vi "测试参数读取.vi"(4 "error in (no error)":errorcluster caption="错误输入（无错误）", 6 "Container State":T5 caption="容器状态", 7 "Display State In":T1={"功能选择"=enum."扫描", "扫描参数"={"+ V"=1.0, "+ Δ V"=0.01, "+ limit I"=0.01, "- V"=1.0, "- Δ V"=0.01, "- limit I"=0.01, "NPLC"=1.0, "模型"=FALSE}, "保持时间"={"V"=0.1, "limit I"=0.01, "T"=10000.0, "ΔT"=1.0, "NPLC"=1.0}, "脉冲1"={"t0"=timestamp(0 s since 1904-01-01), "dt"=1.0, "Y"=[]}, "脉冲2"={"t0"=timestamp(0 s since 1904-01-01), "dt"=1.0, "Y"=[]}, "高速脉冲1"={"t0"=timestamp(0 s since 1904-01-01), "dt"=1.0, "Y"=[]}, "高速脉冲2"={"t0"=timestamp(0 s since 1904-01-01), "dt"=1.0, "Y"=[]}, "任意波形"={"t0"=timestamp(0 s since 1904-01-01), "dt"=1.0, "Y"=[]}} caption="显示状态输入" {"保持时间"."ΔT" min=0.5 max=100.0 step=0.1 format="%#_6ps"; "保持时间"."T" min=10.0 max=4294000.0 step=1.0 format="%#_6ps"; "保持时间"."NPLC" min=1.0 max=20.0 step=1.0; "保持时间"."limit I" min=1e-08 max=3.0 format="%#_6pA"; "保持时间"."V" min=-40.0 max=40.0 format="%#_6pV"; "扫描参数"."NPLC" min=0.001 max=25.0 step=0.001; "扫描参数"."- Δ V" min=5e-05 max=1.0 step=5e-05 format="%#_6pV"; "扫描参数"."+ Δ V" min=5e-05 max=1.0 step=5e-05 format="%#_6pV"; "扫描参数"."- V" min=-40.0 max=40.0 format="%#_6pV"; "扫描参数"."- limit I" min=1e-08 max=3.0 format="%#_6pA"; "扫描参数"."+ limit I" min=1e-08 max=3.0 format="%#_6pA"; "扫描参数"."+ V" min=-40.0 max=40.0 format="%#_6pV"}) -> (0 "error out":errorcluster caption="错误输出", 2 "Value":variant caption="值", 3 "Display State Out":T1={"功能选择"=enum."扫描", "扫描参数"={"+ V"=1.0, "+ Δ V"=0.01, "+ limit I"=0.01, "- V"=1.0, "- Δ V"=0.01, "- limit I"=0.01, "NPLC"=1.0, "模型"=FALSE}, "保持时间"={"V"=0.1, "limit I"=0.01, "T"=10000.0, "ΔT"=1.0, "NPLC"=1.0}, "脉冲1"={"t0"=timestamp(0 s since 1904-01-01), "dt"=1.0, "Y"=[]}, "脉冲2"={"t0"=timestamp(0 s since 1904-01-01), "dt"=1.0, "Y"=[]}, "高速脉冲1"={"t0"=timestamp(0 s since 1904-01-01), "dt"=1.0, "Y"=[]}, "高速脉冲2"={"t0"=timestamp(0 s since 1904-01-01), "dt"=1.0, "Y"=[]}, "任意波形"={"t0"=timestamp(0 s since 1904-01-01), "dt"=1.0, "Y"=[]}} caption="显示状态输出" {"保持时间"."ΔT" min=0.5 max=100.0 step=0.1 format="%#_6ps"; "保持时间"."T" min=10.0 max=4294000.0 step=1.0 format="%#_6ps"; "保持时间"."NPLC" min=1.0 max=20.0 step=1.0; "保持时间"."limit I" min=1e-08 max=3.0 format="%#_6pA"; "保持时间"."V" min=-40.0 max=40.0 format="%#_6pV"; "扫描参数"."NPLC" min=0.001 max=25.0 step=0.001; "扫描参数"."- Δ V" min=5e-05 max=1.0 step=5e-05 format="%#_6pV"; "扫描参数"."+ Δ V" min=5e-05 max=1.0 step=5e-05 format="%#_6pV"; "扫描参数"."- V" min=-40.0 max=40.0 format="%#_6pV"; "扫描参数"."- limit I" min=1e-08 max=3.0 format="%#_6pA"; "扫描参数"."+ limit I" min=1e-08 max=3.0 format="%#_6pA"; "扫描参数"."+ V" min=-40.0 max=40.0 format="%#_6pV"})   [LabVIEW 2020, in "功能选择.xctl"]
uses:
  <vilib>/_xctls/Container State.ctl
  <vilib>/_xctls/XControlSupport.lvlib
panel:
  # "将以下值显示控件替换为所需类型的显示控件。\n不要从连线板中删除该显示控件或其它显示控件。\n不要更改连线板模式。\n值显示控件应始终位于连线板输出端自顶部起第二个接线端。"
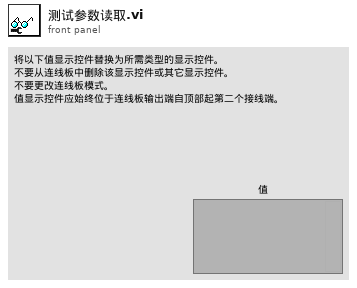
[diagram p1: front panel]
types:
  T1 = typedef "功能选择.xctl/状态.ctl" = cluster{"功能选择":T2, "扫描参数":T3, "保持时间":T4, "脉冲1":waveform(dbl), "脉冲2":waveform(dbl), "高速脉冲1":waveform(dbl), "高速脉冲2":waveform(dbl), "任意波形":waveform(dbl)}
  T2 = typedef "功能选择.xctl/功能类型选择.ctl" = enum16{"扫描", "循环扫描", "保持时间", "脉冲", "高速脉冲", "任意波形"}
  T3 = typedef "功能选择.xctl/扫描参数.ctl" = cluster{"+ V":dbl, "+ Δ V":dbl, "+ limit I":dbl, "- V":dbl, "- Δ V":dbl, "- limit I":dbl, "NPLC":dbl, "模型":bool}
  T4 = typedef "功能选择.xctl/保持时间.ctl" = cluster{"V":dbl, "limit I":dbl, "T":dbl, "ΔT":dbl, "NPLC":dbl}
  T5 = typedef "XControlSupport.lvlib/Container State.ctl" = cluster{"Indicator?":bool, "Run Mode?":bool, " Refnum":refnum<vi>}
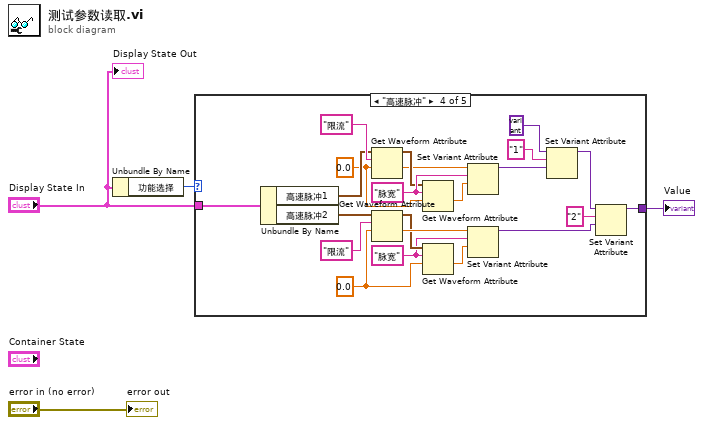
[diagram p0: block diagram]
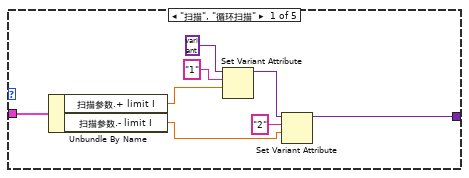
[diagram p2: hidden frame]
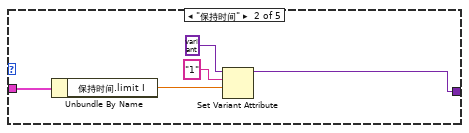
[diagram p3: hidden frame]
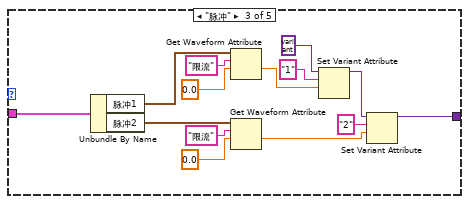
[diagram p4: hidden frame]
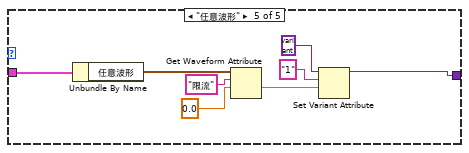
[diagram p5: hidden frame]
diagram:
  n1 = Unbundle By Name("Display State In") -> ("功能选择"=w3:T2)
  n2 = case shown="\"高速脉冲\"" w3 {
    tunnel: "Display State In" -> [w12 w17 w31 w53 w61]
    tunnel: [w5 w13 w27 w49 w54] -> w1
    frame "扫描", "循环扫描" {
      n3 = Unbundle By Name(w12) -> ("扫描参数.+ limit I"=w10:dbl, "扫描参数.- limit I"=w8:dbl)
      n4 = Set Variant Attribute(Variant=variant ("变体"), name="1" ("名称"), value=w10) -> (Variant out=w7:variant)  [unwired: 1 in, 2 out]
      n5 = Set Variant Attribute(Variant=w7, name="2" ("名称"), value=w8) -> (Variant out=w5:variant)  [unwired: 1 in, 2 out]
    }
    frame "保持时间" {
      n6 = Unbundle By Name(w17) -> ("保持时间.limit I"=w14:dbl)
      n7 = Set Variant Attribute(Variant=variant ("变体"), name="1" ("名称"), value=w14) -> (Variant out=w13:variant)  [unwired: 1 in, 2 out]
    }
    frame "脉冲" {
      n8 = Unbundle By Name(w31) -> ("脉冲1"=w25:waveform(dbl), "脉冲2"=w19:waveform(dbl))
      n9 = Get Waveform Attribute(5:0.0, 6:"限流" ("名称"), 7:w25) -> (1:w22:dbl)  [unwired: 1 in, 3 out]
      n10 = Get Waveform Attribute(5:0.0, 6:"限流" ("名称"), 7:w19) -> (1:w18:dbl)  [unwired: 1 in, 3 out]
      n11 = Set Variant Attribute(Variant=variant ("变体"), name="1" ("名称"), value=w22) -> (Variant out=w28:variant)  [unwired: 1 in, 2 out]
      n12 = Set Variant Attribute(Variant=w28, name="2" ("名称"), value=w18) -> (Variant out=w27:variant)  [unwired: 1 in, 2 out]
    }
    frame "高速脉冲" {
      w32 = 0.0
      w40 = "脉宽" ("名称")
      w33 = 0.0
      w41 = "脉宽" ("名称")
      n13 = Unbundle By Name(w53) -> ("高速脉冲1"=w35:waveform(dbl), "高速脉冲2"=w46:waveform(dbl))
      n14 = Get Waveform Attribute(5:w32, 6:"限流" ("名称"), 7:w35) -> (1:w37:dbl, 3:w38:waveform(dbl))  [unwired: 1 in, 2 out]
      n15 = Get Waveform Attribute(5:w33, 6:"限流" ("名称"), 7:w46) -> (1:w45:dbl, 3:w43:waveform(dbl))  [unwired: 1 in, 2 out]
      n16 = Get Waveform Attribute(5:w32, 6:w40, 7:w38) -> (1:w39:dbl)  [unwired: 1 in, 3 out]
      n17 = Get Waveform Attribute(5:w33, 6:w41, 7:w43) -> (1:w42:dbl)  [unwired: 1 in, 3 out]
      n18 = Set Variant Attribute(Variant=w37, name=w40, value=w39) -> (Variant out=w34:variant)  [unwired: 1 in, 2 out]
      n19 = Set Variant Attribute(Variant=w45, name=w41, value=w42) -> (Variant out=w44:variant)  [unwired: 1 in, 2 out]
      n20 = Set Variant Attribute(Variant=variant ("变体"), name="1" ("名称"), value=w34) -> (Variant out=w50:variant)  [unwired: 1 in, 2 out]
      n21 = Set Variant Attribute(Variant=w50, name="2" ("名称"), value=w44) -> (Variant out=w49:variant)  [unwired: 1 in, 2 out]
    }
    frame "任意波形" {
      n22 = Unbundle By Name(w61) -> ("任意波形"=w55:waveform(dbl))
      n23 = Get Waveform Attribute(5:0.0, 6:"限流" ("名称"), 7:w55) -> (1:w56:dbl)  [unwired: 1 in, 3 out]
      n24 = Set Variant Attribute(Variant=variant ("变体"), name="1" ("名称"), value=w56) -> (Variant out=w54:variant)  [unwired: 1 in, 2 out]
    }
  }
  "Value" <- w1
  "error out" <- "error in (no error)"
  "Display State Out" <- "Display State In"
